vi "RunDuringExperiment_20May2014.vi"() -> ()   [LabVIEW 2012]
uses:
  GlobalVars.vi
panel:
  in  "Analyze Nth Frames":i32=10 min=1 step=1
  out "Motion Computation Error":errorcluster
  out "Elements in Data Queue":i32
  in  "Position Shift Limit (Microns)":dbl=3.0 min=0.0
  out "Out of Limits":bool
  out "Z1":waveform(dbl)(graph)
  out "Y1":waveform(dbl)(graph)
  out "X1":waveform(dbl)(graph)
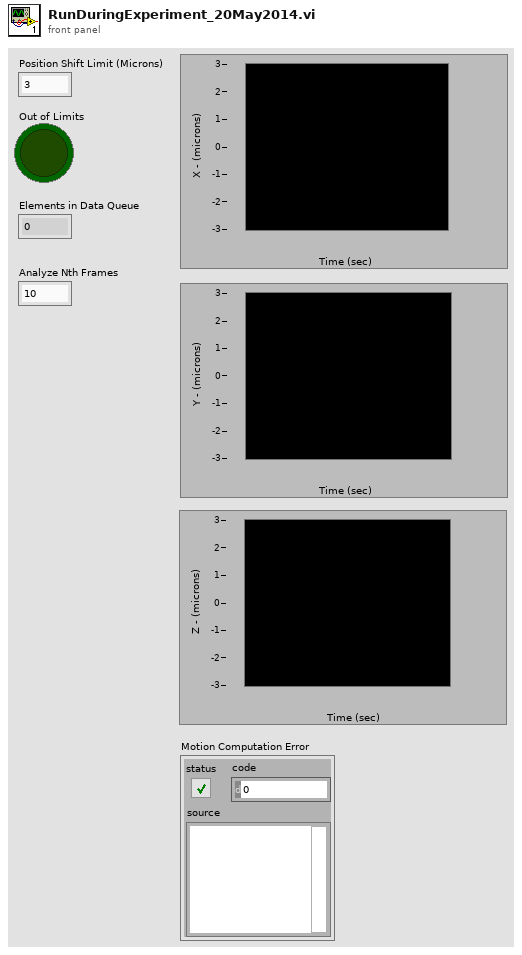
[diagram p1: front panel]
types:
  T1 = cluster{"gridsize":u16, "data":i32[][], "coordinates":i32[][], "settings":i32[], "settings_um":i32[], "needsreference":bool}
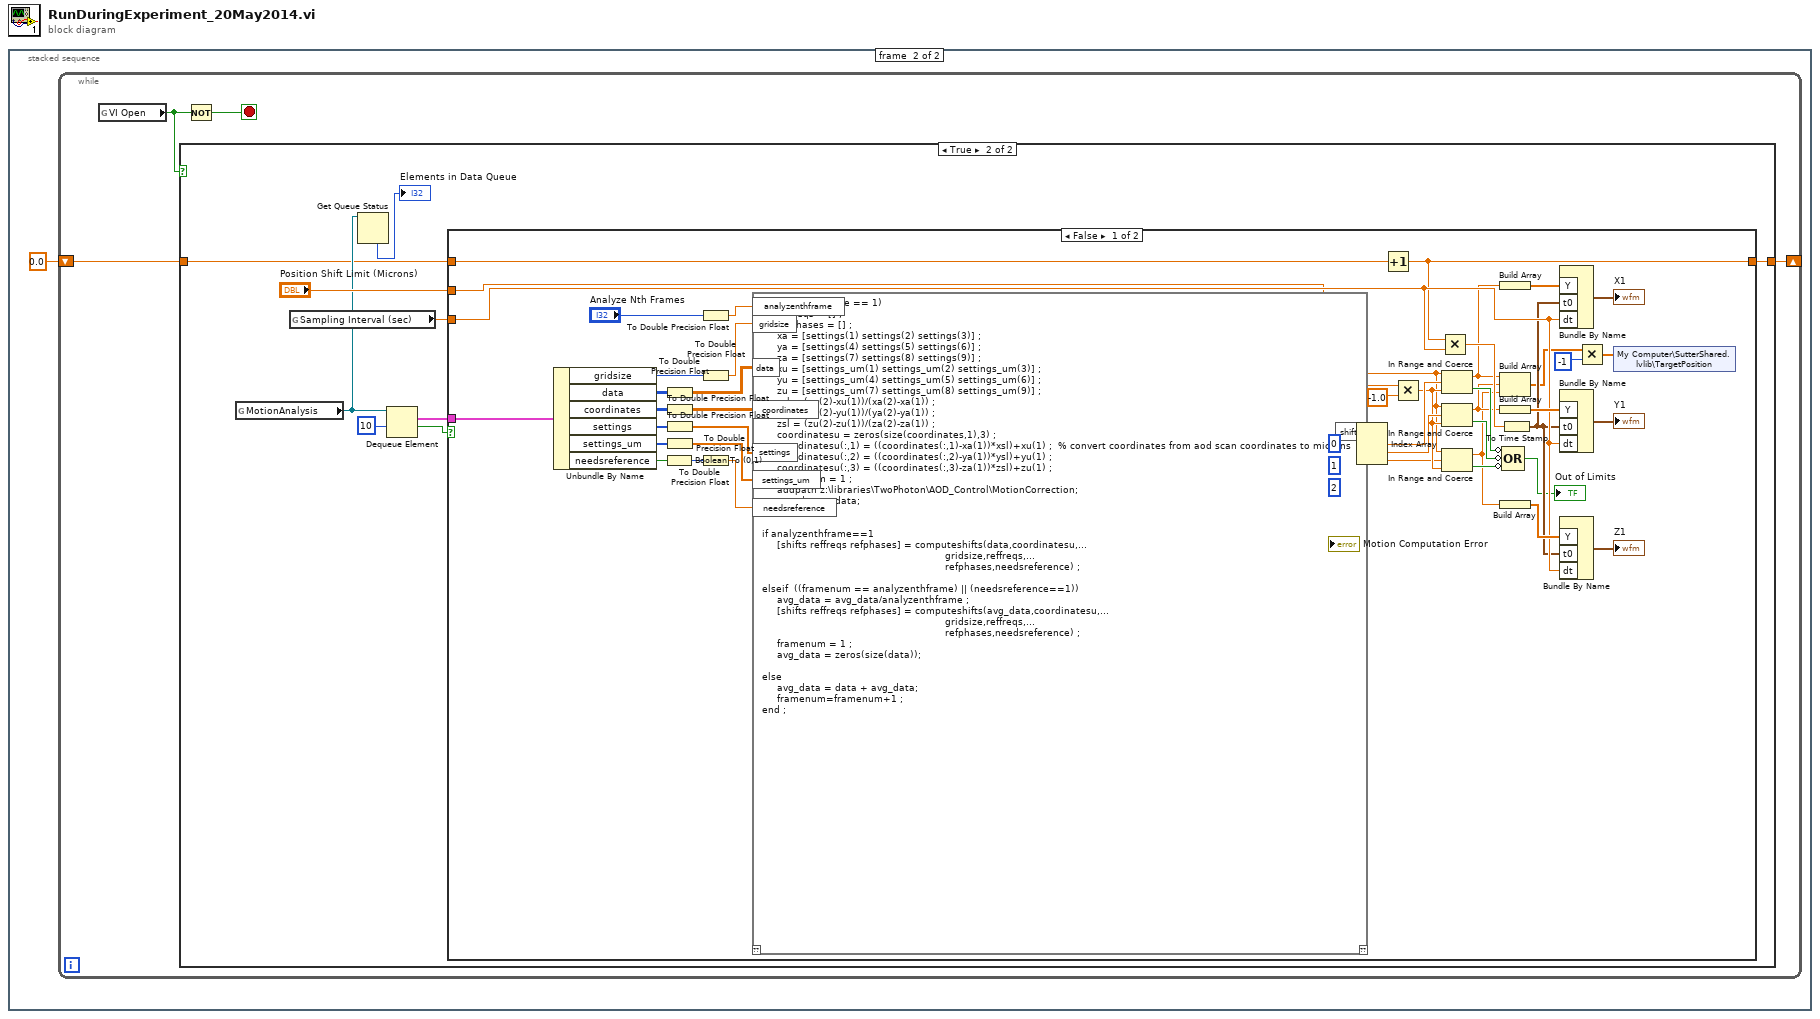
[diagram p0: block diagram]
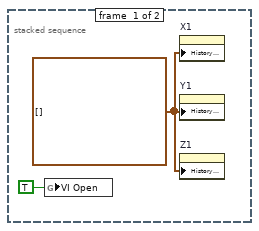
[diagram p2: hidden frame]
diagram:
  n1 = stacked-sequence {
    frame #0 {
      w1 = waveform(dbl)[] [] ("History Data")
      n2 = global write "GlobalVars.vi" "VI Open"(TRUE ("VI Open")) -> ()
      n3 = property on="X1" class="WFChart (strict)"("History Data"=w1) -> ()  [unwired: 2 in, 2 out]
      n4 = property on="Y1" class="WFChart (strict)"("History Data"=w1) -> ()  [unwired: 2 in, 2 out]
      n5 = property on="Z1" class="WFChart (strict)"("History Data"=w1) -> ()  [unwired: 2 in, 2 out]
    }
    frame #1 {
      n6 = while {
        shift-right: [w4] -> _
        shift-left: 0.0 -> [w5]
        stop <- w7 stop-if-true
        n7 = global read "GlobalVars.vi" "VI Open"() -> (w6:bool)
        n8 = case shown="True" w6 {
          tunnel: w5 -> [w8 w11]
          tunnel: [w8 w10] -> w4
          frame False {
          }
          frame True {
            n9 = global read "GlobalVars.vi" "MotionAnalysis"() -> (w13:refnum<queue>)
            n10 = global read "GlobalVars.vi" "Sampling Interval (sec)"() -> (w9:dbl)
            n11 = Get Queue Status(queue=w13) -> (# elements in queue=→"Elements in Data Queue":i32)  [unwired: 2 in, 7 out]
            n12 = Dequeue Element(queue=w13, timeout in ms (-1)=10) -> (element=w16:T1, timed out?=w15:bool)  [unwired: 1 in, 2 out]
            n13 = case shown="False" w15 {
              tunnel: "Position Shift Limit (Microns)" -> [w50 _]
              tunnel: w16 -> [w34 _]
              tunnel: w9 -> [w57 _]
              tunnel: w11 -> [w59 w66]
              tunnel: [w56 w66] -> w10
              frame False {
                n14 = Unbundle By Name(w34) -> ("gridsize"=w33:u16, "data"=w31:i32[][], "coordinates"=w29:i32[][], "settings"=w27:i32[], "settings_um"=w25:i32[], "needsreference"=w21:bool)
                n15 = Boolean To (0,1)(Boolean=w21) -> (0, 1=w22:i16)
                n16 = To Double Precision Float(number=w31) -> (double precision float=w30:dbl[][])
                n17 = To Double Precision Float(number=w29) -> (double precision float=w28:dbl[][])
                n18 = To Double Precision Float(number=w27) -> (double precision float=w26:dbl[])
                n19 = To Double Precision Float(number=w25) -> (double precision float=w24:dbl[])
                n20 = To Double Precision Float(number="Analyze Nth Frames") -> (double precision float=w19:dbl)
                n21 = To Double Precision Float(number=w33) -> (double precision float=w32:dbl)
                n22 = To Double Precision Float(number=w22) -> (double precision float=w23:dbl)
                n23 = script code="if (needsreference == 1)\n     reffreqs = [] ;\n     refphases = [] ;\n     xa = [settings(1) settings(2) settings(3)] ;\n     ya = [settings(4) settings(5) settings(6)] ;\n     za = [settings(7) settings(8) settings(9)] ;\n     xu = [settings_um(1) settings_um(2) settings_um(3)] ;\n     yu = [settings_um(4) settings_um(5) settings_um(6)] ;\n     zu = [settings_um(7) settings_um(8) settings_um(9)] ;\n     xsl = (xu(2)-xu(1))/(xa(2)-xa(1)) ;\n     ysl = (yu(2)-yu(1))/(ya(2)-ya(1)) ;\n     zsl = (zu(2)-zu(1))/(za(2)-za(1)) ;\n     coordinatesu = zeros(size(coordinates,1),3) ;\n     coordinatesu(:,1) = ((coordinates(:,1)-xa(1))*xsl)+xu(1) ;  % convert coordinates from aod scan coordinates to microns\n     coordinatesu(:,2) = ((coordinates(:,2)-ya(1))*ysl)+yu(1) ;\n     coordinatesu(:,3) = ((coordinates(:,3)-za(1))*zsl)+zu(1) ;\n     framenum = 1 ;\n     addpath z:\\libraries\\TwoPhoton\\AOD_Control\\MotionCorrection;\n     avg_data = data;\nend\n\nif analyzenthframe==1\n     [shifts reffreqs refphases] = computeshifts(data,coordinatesu,...\n                                                             gridsize,reffreqs,...\n                                                             refphases,needsreference) ; \n\nelseif  ((framenum == analyzenthframe) || (needsreference==1))\n     avg_data = avg_data/analyzenthframe ;\n     [shifts reffreqs refphases] = computeshifts(avg_data,coordinatesu,...\n                                                             gridsize,reffreqs,...\n                                                             refphases,needsreference) ; \n     framenum = 1 ;\n     avg_data = zeros(size(data));\n\nelse\n     avg_data = data + avg_data;\n     framenum=framenum+1 ;\nend ;"("data"=w30, "coordinates"=w28, "gridsize"=w32, "needsreference"=w23, "settings"=w26, "settings_um"=w24, "analyzenthframe"=w19) -> ("??"=→"Motion Computation Error":errorcluster, "shifts"=w35:dbl[])  [unwired: 1 in]
                n24 = Index Array(array=w35, index #1=0 ("index"), index #2=1 ("index"), index #3=2 ("index")) -> (element #1=w53:dbl, element #2=w52:dbl, element #3=w49:dbl)
                n25 = Increment(x=w59) -> (x+1=w56:dbl)
                n26 = Multiply(x=w50, y=-1.0) -> (x*y=w51:dbl)
                n27 = Multiply(x=w56, y=w57) -> (x*y=w58:dbl)
                n28 = In Range and Coerce(upper limit=w50, x=w53, lower limit=w51) -> (coerced(x)=w44:dbl, In Range?=w48:bool)
                n29 = In Range and Coerce(upper limit=w50, x=w52, lower limit=w51) -> (coerced(x)=w43:dbl, In Range?=w47:bool)
                n30 = In Range and Coerce(upper limit=w50, x=w49, lower limit=w51) -> (coerced(x)=w42:dbl, In Range?=w46:bool)
                n31 = Build Array(w44) -> (w64:dbl[])
                n32 = Build Array(w44, w43, w42) -> (w41:dbl[])
                n33 = Build Array(w43) -> (w60:dbl[])
                n34 = Build Array(w42) -> (w61:dbl[])
                n35 = To Time Stamp(1:w58) -> (0:w55:timestamp)
                n36 = Compound Arithmetic op=OR(invert w48, invert w47, invert w46) -> (→"Out of Limits":bool)
                n37 = Bundle By Name("Y"=w64, "t0"=w55, "dt"=w57) -> (→"X1":waveform(dbl))  [unwired: 1 in]
                n38 = Bundle By Name("Y"=w60, "t0"=w55, "dt"=w57) -> (→"Y1":waveform(dbl))  [unwired: 1 in]
                n39 = Bundle By Name("Y"=w61, "t0"=w55, "dt"=w57) -> (→"Z1":waveform(dbl))  [unwired: 1 in]
                n40 = Multiply(x=w41, y=-1) -> (x*y=w39:dbl[])
                n41 = shared-variable "My Computer\\SutterShared.lvlib\\TargetPosition"(w39) -> ()  [unwired: 1 in, 1 out]
              }
              frame True {
              }
            }
          }
        }
        n42 = Not(x=w6) -> (.not. x?=w7:bool)
      }
    }
  }
